vi "S2C_PCIe7841_Proc_AnalogRead.vi"(8 "Error In":errorcluster, 11 "Data":string) -> (0 "Error Out":errorcluster, 3 "Result":string)   [LabVIEW 2015]
uses:
  S2C_PCIe7841_Proc_Globals.vi
  <vilib>/Utility/error.llb/Error Cluster From Error Code.vi
  <vilib>/rvi/errors/niLvFpgaAdjustHostInterfaceError.vi
  <vilib>/rvi/interface/nirviReadWriteControl/nirviReadWriteControl.xnode
  <vilib>/rvi/interface/Simulation/niFpgaSimulationCallBeginRW.vi
  NiFpgaLv.dll
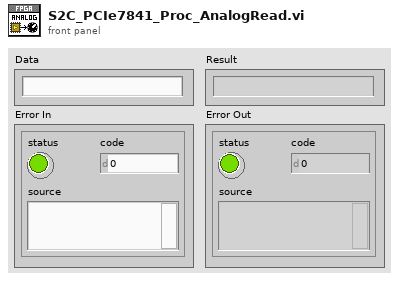
[diagram p1: front panel]
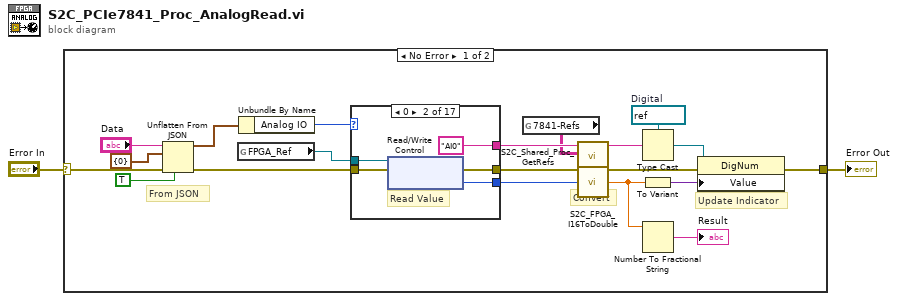
[diagram p0: block diagram]
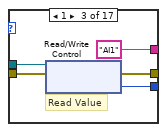
[diagram p3: hidden frame]
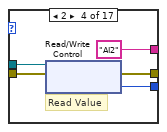
[diagram p4: hidden frame]
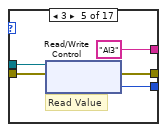
[diagram p5: hidden frame]
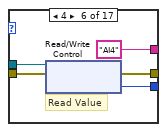
[diagram p6: hidden frame]
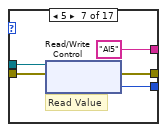
[diagram p7: hidden frame]
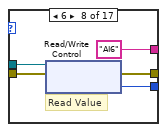
[diagram p8: hidden frame]
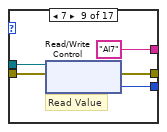
[diagram p9: hidden frame]
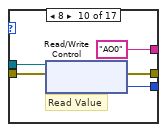
[diagram p10: hidden frame]
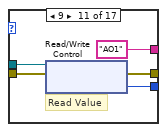
[diagram p11: hidden frame]
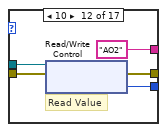
[diagram p12: hidden frame]
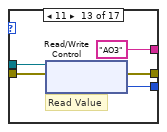
[diagram p13: hidden frame]
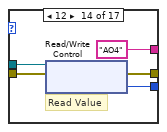
[diagram p14: hidden frame]
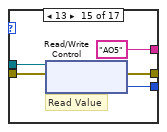
[diagram p15: hidden frame]
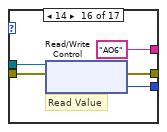
[diagram p16: hidden frame]
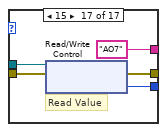
[diagram p17: hidden frame]
diagram:
  n1 = case shown="No Error" "Error In" {
    selector: "Error In" -> [w22 w104]
    tunnel: [w8 w104] -> w1
    frame No Error {
      w13 = refnum<vi> refnum  # Digital
      # "Convert"
      # "Update Indicator"
      # "From JSON"
      n2 = Unflatten From JSON(JSON string="Data", type and defaults=cluster{"Analog IO":u16} {"Analog IO"=0}, default null elements? (F)=TRUE, error in (no error)=w22) -> (value=w19:cluster{"Analog IO":u16}, error out=w17:errorcluster)  [unwired: 3 in]
      n3 = global read "S2C_PCIe7841_Proc_Globals.vi" "FPGA_Ref"() -> (w16:refnum<k20>)
      n4 = Unbundle By Name(w19) -> ("Analog IO"=w18:u16)
      n5 = case shown="0" w18 {
        tunnel: w17 -> [w23 w28 w33 w38 w43 w48 w53 w58 w63 w68 w73 w78 w83 w88 w93 w98 w103]
        tunnel: w16 -> [_ w27 w32 w37 w42 w47 w52 w57 w62 w67 w72 w77 w82 w87 w92 w97 w102]
        tunnel: [w23 w26 w31 w36 w41 w46 w51 w56 w61 w66 w71 w76 w81 w86 w91 w96 w101] -> w9
        tunnel: [_ w25 w30 w35 w40 w45 w50 w55 w60 w65 w70 w75 w80 w85 w90 w95 w100] -> w14
        tunnel: [_ "AI0" ("Label") "AI1" ("Label") "AI2" ("Label") "AI3" ("Label") "AI4" ("Label") "AI5" ("Label") "AI6" ("Label") "AI7" ("Label") "AO0" ("Label") "AO1" ("Label") "AO2" ("Label") "AO3" ("Label") "AO4" ("Label") "AO5" ("Label") "AO6" ("Label") "AO7" ("Label")] -> w7
        frame 16, Default {
        }
        frame 0 {
          # "Read Value"
          n6 = xnode "Read/Write Control"("FPGA VI Reference In"=w27, "error in"=w28) -> ("error out"=w26:errorcluster, "Conn0/AI0"=w25:i16)  [unwired: 1 out]
        }
        frame 1 {
          # "Read Value"
          n7 = xnode "Read/Write Control"("FPGA VI Reference In"=w32, "error in"=w33) -> ("error out"=w31:errorcluster, "Conn0/AI1"=w30:i16)  [unwired: 1 out]
        }
        frame 2 {
          # "Read Value"
          n8 = xnode "Read/Write Control"("FPGA VI Reference In"=w37, "error in"=w38) -> ("error out"=w36:errorcluster, "Conn0/AI2"=w35:i16)  [unwired: 1 out]
        }
        frame 3 {
          # "Read Value"
          n9 = xnode "Read/Write Control"("FPGA VI Reference In"=w42, "error in"=w43) -> ("error out"=w41:errorcluster, "Conn0/AI3"=w40:i16)  [unwired: 1 out]
        }
        frame 4 {
          # "Read Value"
          n10 = xnode "Read/Write Control"("FPGA VI Reference In"=w47, "error in"=w48) -> ("error out"=w46:errorcluster, "Conn0/AI4"=w45:i16)  [unwired: 1 out]
        }
        frame 5 {
          # "Read Value"
          n11 = xnode "Read/Write Control"("FPGA VI Reference In"=w52, "error in"=w53) -> ("error out"=w51:errorcluster, "Conn0/AI5"=w50:i16)  [unwired: 1 out]
        }
        frame 6 {
          # "Read Value"
          n12 = xnode "Read/Write Control"("FPGA VI Reference In"=w57, "error in"=w58) -> ("error out"=w56:errorcluster, "Conn0/AI6"=w55:i16)  [unwired: 1 out]
        }
        frame 7 {
          # "Read Value"
          n13 = xnode "Read/Write Control"("FPGA VI Reference In"=w62, "error in"=w63) -> ("error out"=w61:errorcluster, "Conn0/AI7"=w60:i16)  [unwired: 1 out]
        }
        frame 8 {
          # "Read Value"
          n14 = xnode "Read/Write Control"("FPGA VI Reference In"=w67, "error in"=w68) -> ("error out"=w66:errorcluster, "Conn0/AO0"=w65:i16)  [unwired: 1 out]
        }
        frame 9 {
          # "Read Value"
          n15 = xnode "Read/Write Control"("FPGA VI Reference In"=w72, "error in"=w73) -> ("error out"=w71:errorcluster, "Conn0/AO1"=w70:i16)  [unwired: 1 out]
        }
        frame 10 {
          # "Read Value"
          n16 = xnode "Read/Write Control"("FPGA VI Reference In"=w77, "error in"=w78) -> ("error out"=w76:errorcluster, "Conn0/AO2"=w75:i16)  [unwired: 1 out]
        }
        frame 11 {
          # "Read Value"
          n17 = xnode "Read/Write Control"("FPGA VI Reference In"=w82, "error in"=w83) -> ("error out"=w81:errorcluster, "Conn0/AO3"=w80:i16)  [unwired: 1 out]
        }
        frame 12 {
          # "Read Value"
          n18 = xnode "Read/Write Control"("FPGA VI Reference In"=w87, "error in"=w88) -> ("error out"=w86:errorcluster, "Conn0/AO4"=w85:i16)  [unwired: 1 out]
        }
        frame 13 {
          # "Read Value"
          n19 = xnode "Read/Write Control"("FPGA VI Reference In"=w92, "error in"=w93) -> ("error out"=w91:errorcluster, "Conn0/AO5"=w90:i16)  [unwired: 1 out]
        }
        frame 14 {
          # "Read Value"
          n20 = xnode "Read/Write Control"("FPGA VI Reference In"=w97, "error in"=w98) -> ("error out"=w96:errorcluster, "Conn0/AO6"=w95:i16)  [unwired: 1 out]
        }
        frame 15 {
          # "Read Value"
          n21 = xnode "Read/Write Control"("FPGA VI Reference In"=w102, "error in"=w103) -> ("error out"=w101:errorcluster, "Conn0/AO7"=w100:i16)  [unwired: 1 out]
        }
      }
      n22 = global read "S2C_PCIe7841_Proc_Globals.vi" "7841-Refs"() -> (w6:string[][])
      n23 = call "S2C_Shared_Proc_GetRefs.vi"("Error In"=w9, "Refs"=w6, "Label"=w7) -> ("Error Out"=w10:errorcluster, "Reference"=w12:string)  [unwired: 7 in]
      n24 = call "S2C_FPGA_I16ToDouble.vi"("I16 In"=w14) -> ("Double Out"=w4:dbl)  [unwired: 4 in]
      n25 = Type Cast(type=w13, x=w12) -> (*(type *) &x=w11:refnum<vi>)
      n26 = To Variant(anything=w4) -> (Variant=w5:variant)
      n27 = Number To Fractional String(number=w4) -> (F-format string=→"Result":string)  [unwired: 3 in]
      n28 = property class="DigNum"(reference=w11, error in=w10, "Value"=w5) -> (error out=w8:errorcluster)  [unwired: 1 out]
    }
    frame Error {
    }
  }
  "Error Out" <- w1
